vi "Event Messenger Channel Lesson 2.vi"() -> ()   [LabVIEW 2023]
doc: "Lesson 2 shows how multiple Event Messenger channel wires of different data types can both write to the same Event structure."
uses:
  <extravilib>/ChannelInstances/Event Messenger-i32/Event Data.ctl
  <extravilib>/ChannelInstances/Event Messenger-str/Event Data.ctl
  <extravilib>/ChannelInstances/Event Messenger-i32/Instantiate.vi
  <extravilib>/ChannelInstances/Event Messenger-i32/))Channel.vi
  <extravilib>/ChannelInstances/Event Messenger-str/Instantiate.vi
  <extravilib>/ChannelInstances/Event Messenger-str/))Channel.vi
  <extravilib>/ChannelInstances/Event Messenger-i32.lvlib
  <extravilib>/ChannelInstances/Event Messenger-str.lvlib
panel:
  out "Producer Hex":string="0"
  out "Producer Decimal":i32
  out "Number of times clicked":i32
  in  "Click Me":bool
  out "Consumer Hex":string="0"
  in  "Stop Hex":bool
  out "Consumer Decimal":i32
  in  "Stop Decimal":bool
  # "Overview: This VI demonstrates how to use the Event Messenger channel wire.\n\nLesson 2 shows how multiple Event Messenger channel wires of different data types can both write to the same Event structure.\n\n\nInstructions:\n1. Run the VI. Notice that both Producers run faster than the Consumer and at different speeds from each other.\n2. While the VI is running, press the Click Me button. Each time you do, the counter will be incremented.\n3. Stop the VI by hitting one and then the other of the two Stop buttons. You can press them in either order.\n4. Open the block diagram. Review the comments there to see how this VI works."
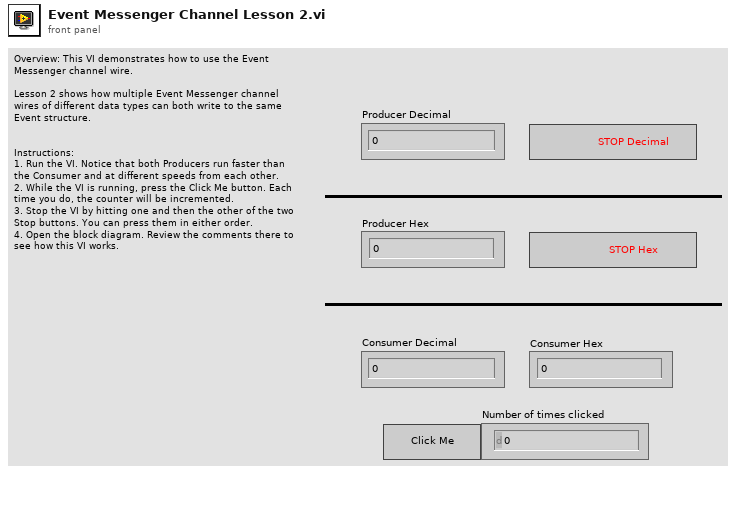
[diagram p1: front panel]
types:
  T1 = cluster{"decimal":refnum<event-registration>, "hex":refnum<event-registration>}
  T2 = typedef "Event Messenger-i32.lvlib/))Channel.ctl" = refnum<queue>
  T3 = typedef "Event Messenger-str.lvlib/))Channel.ctl" = refnum<queue>
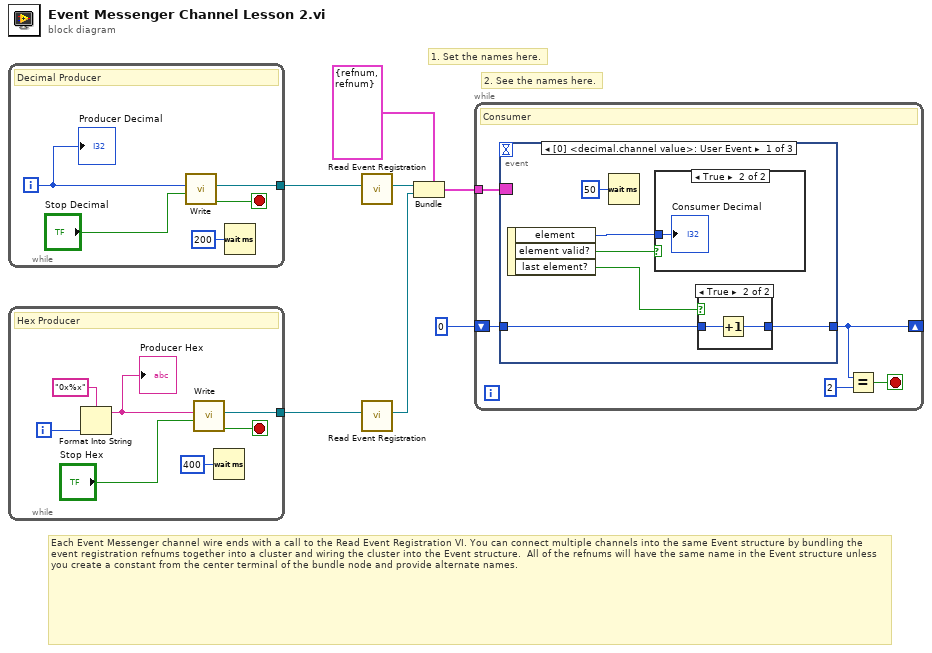
[diagram p0: block diagram]
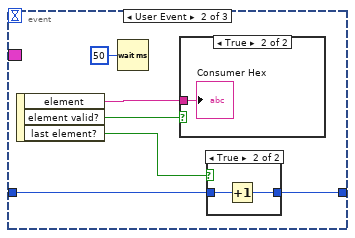
[diagram p4: hidden frame]
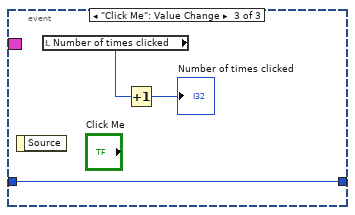
[diagram p7: hidden frame]
diagram:
  # "2. See the names here."
  # "1. Set the names here."
  # "Each Event Messenger channel wire ends with a call to the Read Event Registration VI. You can connect multiple channels into the same Event structure by bundling the event registration refnums together into a cluster and wiring the cluster into the Event structure.  All of the refnums will have the same name in the Event structure unless you create a constant from the center terminal of the bundle node and provide alternate names."
  n1 = while {
    tunnel: [w10] -> w3
    i -> [w8]
    stop <- w12 stop-if-true
    # "Decimal Producer"
    n2 = call <extravilib>:"Write.vi"("last element? (F)"="Stop Decimal", "element"=w8) -> ("done?"=w12:bool, "channel"=w10:T2)  [unwired: 8 in]
    n3 = Wait (ms)(milliseconds to wait=u32 200) -> ()  [unwired: 1 out]
    "Producer Decimal" <- w8
  }
  n4 = while {
    tunnel: [w17] -> w4
    i -> [w14]
    stop <- w19 stop-if-true
    # "Hex Producer"
    n5 = Format Into String(format string="0x%x", w14) -> (resulting string=w13:string)  [unwired: 2 in, 1 out]
    "Producer Hex" <- w13
    n6 = call <extravilib>:"Write.vi"("last element? (F)"="Stop Hex", "element"=w13) -> ("done?"=w19:bool, "channel"=w17:T3)  [unwired: 8 in]
    n7 = Wait (ms)(milliseconds to wait=u32 400) -> ()  [unwired: 1 out]
  }
  n8 = call <extravilib>:"Read Event Registration.vi"("channel"=w3) -> ("event registration refnum"=w2:refnum<event-registration>)  [unwired: 10 in]
  n9 = call <extravilib>:"Read Event Registration.vi"("channel"=w4) -> ("event registration refnum"=w1:refnum<event-registration>)  [unwired: 10 in]
  n10 = Bundle(cluster=T1 {"decimal"=refnum, "hex"=refnum}, "decimal"=w2, "hex"=w1) -> (w7:T1)
  n11 = while {
    tunnel: w7 -> [w24]
    shift-right: [w22] -> _
    shift-left: 0 -> [w23]
    stop <- w20 stop-if-true
    # "Consumer"
    n12 = event shown="[0] <decimal.channel value>: User Event" {
      selector: w24 -> [_ _ _]
      dyn-events: _ -> [_ _ _]
      timeout: _ -> [_ _ _]
      tunnel: w23 -> [w27 w37 w45]
      tunnel: [w26 w36 w45] -> w22
      event User Event {
        n13 = event-data() -> ("element"=w30:i32, "element valid?"=w29:bool, "last element?"=w25:bool)  [unwired: 1 in]
        n14 = Wait (ms)(milliseconds to wait=u32 50) -> ()  [unwired: 1 out]
        n15 = case shown="True" w29 {
          tunnel: w30 -> [_ w34]
          frame False {
          }
          frame True {
            "Consumer Decimal" <- w34
          }
        }
        n16 = case shown="True" w25 {
          tunnel: w27 -> [w31 w33]
          tunnel: [w31 w32] -> w26
          frame False {
          }
          frame True {
            n17 = Increment(x=w33) -> (x+1=w32:i32)
          }
        }
      }
      event User Event {
        n18 = event-data() -> ("element"=w40:string, "element valid?"=w39:bool, "last element?"=w35:bool)  [unwired: 1 in]
        n19 = Wait (ms)(milliseconds to wait=u32 50) -> ()  [unwired: 1 out]
        n20 = case shown="True" w39 {
          tunnel: w40 -> [_ w44]
          frame False {
          }
          frame True {
            "Consumer Hex" <- w44
          }
        }
        n21 = case shown="True" w35 {
          tunnel: w37 -> [w41 w43]
          tunnel: [w41 w42] -> w36
          frame False {
          }
          frame True {
            n22 = Increment(x=w43) -> (x+1=w42:i32)
          }
        }
      }
      event "Click Me": Value Change {
        n23 = event-data() -> ()  [unwired: 1 in, 1 out]
        n24 = local read "Number of times clicked"() -> (w46:i32)
        n25 = Increment(x=w46) -> (x+1=→"Number of times clicked":i32)
      }
    }
    n26 = Equal?(x=w22, y=2) -> (x = y?=w20:bool)
  }
